vi "Initialize.vi"(8 "error in (no error)":errorcluster, 9 "Reset (True)":bool=TRUE, 10 "ID Query (True)":bool=TRUE, 11 "VISA resource name":refnum<visa-resource-name>) -> (0 "error out":errorcluster, 3 "VISA resource name out":refnum<visa-resource-name>)   [LabVIEW 2016, in "Tektronix AFG 1000 Series.lvlib"]
doc: "Establishes communication with the instrument and optionally performs an instrument identification query and/or an instrument reset. It also places the instrument in a default state needed for other instrument driver operations. Therefore, call this VI before calling other instrument driver VIs for this instrument. Generally, you need to call the <B>Initialize VI</B> only once at the beginning of an application."
uses:
  Tektronix AFG 1000 Series.lvlib
panel:
  # "(c) 2016 National Instruments.  ALL RIGHTS RESERVED."
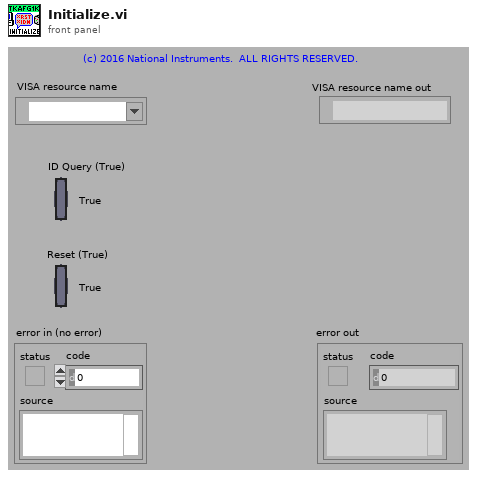
[diagram p1: front panel]
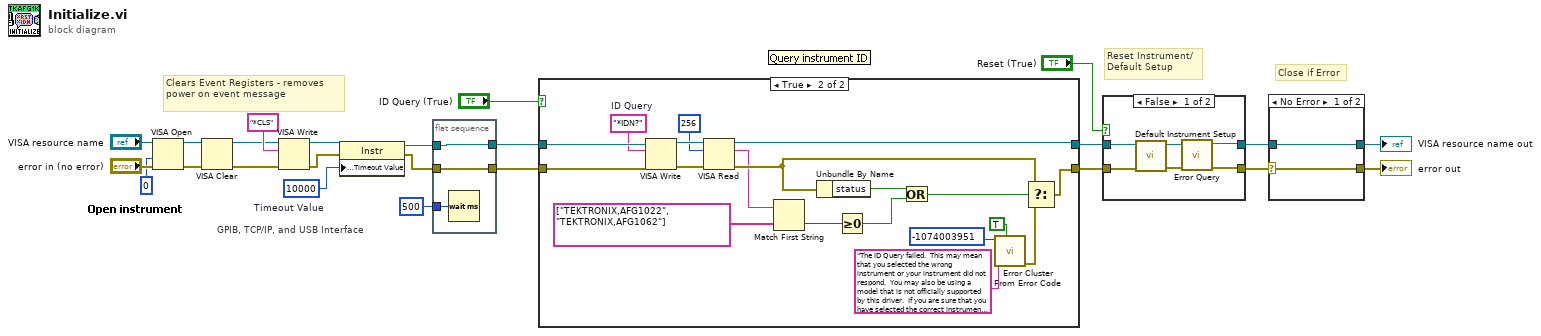
[diagram p0: block diagram]
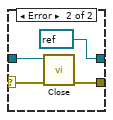
[diagram p2: hidden frame]
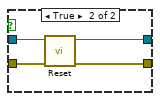
[diagram p3: hidden frame]
diagram:
  w11 = u32 10000  # Timeout Value
  # "Clears Event Registers - removes power on event message"
  # "GPIB, TCP/IP, and USB Interface"
  # "Close if Error"
  # "Reset Instrument/\nDefault Setup"
  n1 = VISA Open(access mode=u32 0, error in (no error)="error in (no error)", VISA resource name="VISA resource name") -> (VISA resource name=w19:refnum<visa-resource-name>, error out=w18:errorcluster)  [unwired: 2 in]
  n2 = VISA Clear(VISA resource name=w19, error in (no error)=w18) -> (VISA resource name out=w9:refnum<visa-resource-name>, error out=w8:errorcluster)
  n3 = VISA Write(VISA resource name=w9, write buffer="*CLS", error in (no error)=w8) -> (VISA resource name out=w7:refnum<visa-resource-name>, error out=w6:errorcluster)  [unwired: 1 out]
  n4 = property class="Instr"(reference=w7, error in=w6, "General Settings:Timeout Value"=w11) -> (reference out=w5:refnum<visa-resource-name>, error out=w3:errorcluster)
  n5 = flat-sequence {
    tunnel: w5 -> [w27]
    tunnel: [w27] -> w4
    tunnel: w3 -> [w26]
    tunnel: [w26] -> w2
    tunnel: u32 500 ("milliseconds to wait") -> [w25]
    frame #0 {
      n6 = Wait (ms)(milliseconds to wait=w25) -> ()  [unwired: 1 out]
    }
  }
  n7 = case shown="True" "ID Query (True)" {
    tunnel: [w28 w37] -> w12
    tunnel: [w29 w46] -> w13
    tunnel: w4 -> [w29 w47]
    tunnel: w2 -> [w28 w48]
    frame False {
    }
    frame True {
      w42 = "*IDN?"  # ID Query
      n8 = VISA Write(VISA resource name=w47, write buffer=w42, error in (no error)=w48) -> (VISA resource name out=w45:refnum<visa-resource-name>, error out=w44:errorcluster)  [unwired: 1 out]
      n9 = VISA Read(VISA resource name=w45, byte count=u32 256, error in (no error)=w44) -> (VISA resource name out=w46:refnum<visa-resource-name>, read buffer=w36:string, error out=w41:errorcluster)  [unwired: 1 out]
      n10 = Match First String(2:string[] ["TEKTRONIX,AFG1022", "TEKTRONIX,AFG1062"], 3:w36) -> (0:w31:i32)  [unwired: 1 out]
      n11 = Unbundle By Name(w41) -> ("status"=w40:bool)
      n12 = Greater Or Equal To 0?(x=w31) -> (x >= 0?=w39:bool)
      n13 = Or(x=w40, y=w39) -> (x .or. y?=w38:bool)
      n14 = call <vilib>:"Error Cluster From Error Code.vi"("show call chain? (False)"=TRUE, "error message (\"\")"="The ID Query failed.  This may mean that you selected the wrong instrument or your instrument did not respond.  You may also be using a model that is not officially supported by this driver.  If you are sure that you have selected the correct instrument and it is responding, try disabling the ID Query." ("Source (VI Name)"), "error code (0)"=-1074003951 ("Code")) -> ("error out"=w32:errorcluster)  [unwired: 6 in]
      n15 = Select(t=w41, s=w38, f=w32) -> (s? t:f=w37:errorcluster)
    }
  }
  n16 = case shown="False" "Reset (True)" {
    tunnel: [w49 w58] -> w14
    tunnel: w13 -> [w54 w56]
    tunnel: [w51 w57] -> w15
    tunnel: w12 -> [w53 w55]
    frame False {
      n17 = call "Default Instrument Setup.vi"("error in (no error) 2"=w53, "VISA resource name 2"=w54) -> ("error out"=w50:errorcluster, "VISA resource name out"=w52:refnum<visa-resource-name>)  [unwired: 8 in]
      n18 = call "Error Query.vi"("error in (no error)"=w50, "VISA resource name"=w52) -> ("error out"=w49:errorcluster, "VISA resource name out"=w51:refnum<visa-resource-name>)  [unwired: 6 in, 2 out]
    }
    frame True {
      n19 = call "Reset.vi"("error in (no error)"=w55, "VISA resource name"=w56) -> ("error out"=w58:errorcluster, "VISA resource name out"=w57:refnum<visa-resource-name>)  [unwired: 8 in]
    }
  }
  n20 = case shown="No Error" w14 {
    selector: w14 -> [w59 w62]
    tunnel: w15 -> [w60 w63]
    tunnel: [w60 refnum<visa-resource-name> refnum ("VISA resource name out")] -> w17
    tunnel: [w59 w64] -> w16
    frame No Error {
    }
    frame Error {
      n21 = call "Close.vi"("error in (no error)"=w62, "VISA resource name"=w63) -> ("error out"=w64:errorcluster)  [unwired: 9 in]
    }
  }
  "VISA resource name out" <- w17
  "error out" <- w16
